vi "ScanString.vi"(8 "error in (no error)":errorcluster, 10 "String":string, 11 "U8 D Element in":refnum<class "U8 D Element.lvclass">) -> (0 "error out":errorcluster, 3 "U8 D Element out":refnum<class "U8 D Element.lvclass">)   [LabVIEW 2020, in "D Datagrid Library.lvlib" / "U8 D Element.lvclass"]
uses:
  U8 D Element.lvclass
  U8 D Element.lvclass/U8 D Element.ctl
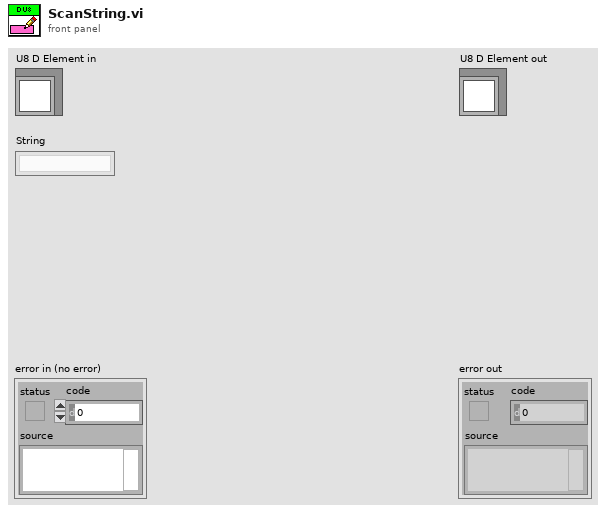
[diagram p1: front panel]
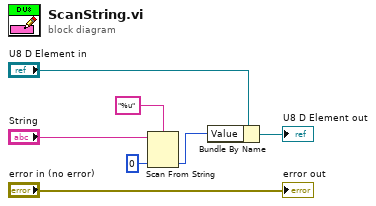
[diagram p0: block diagram]
diagram:
  n1 = Scan From String(format string="%u", input string="String", default 1=u8 0 ("default value 1")) -> (output 1=w3:u8)  [unwired: 2 in, 3 out]
  n2 = Bundle By Name(cluster="U8 D Element in", "Value"=w3) -> (→"U8 D Element out":refnum<class "U8 D Element.lvclass">)
  "error out" <- "error in (no error)"
